vi "globalVariables.vi"() -> ()   [LabVIEW 2020]
panel:
  in  "stop":bool
  out "System user":string
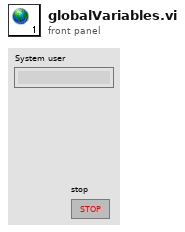
[diagram p1: front panel]
diagram:
